vi "SIM Set Node Final Step Only.vi"(8 "error in (no error)":errorcluster, 11 "node ref":refnum<vi>) -> (0 "error out":errorcluster, 2 "succeeded":bool, 3 "dup node ref":refnum<vi>)   [LabVIEW 2020]
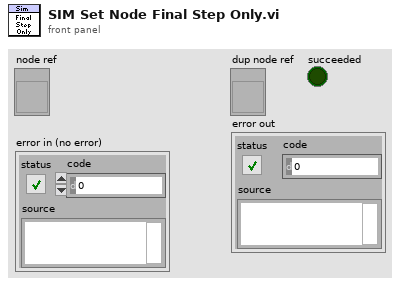
[diagram p1: front panel]
types:
  T1 = enum16{"Function call", "Discrete", "Continuous", "Initialization only", "Final step only"}
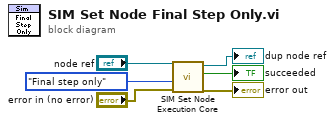
[diagram p0: block diagram]
diagram:
  n1 = call <vilib>:"SIM Set Node Execution Core.vi"("error in (no error)"="error in (no error)", "execution type (continuous)"=T1."Final step only", "Node in"="node ref") -> ("error out"=→"error out":errorcluster, "succeeded"=→"succeeded":bool, "Node out"=→"dup node ref":refnum<vi>)  [unwired: 6 in]
